vi "ClientAPI Tree.vi"   [LabVIEW 2020, in "CSM-TCP-Router.lvlib"]
uses:
  CSM-TCP-Router.lvlib
  TcpRouter-Client.lvclass
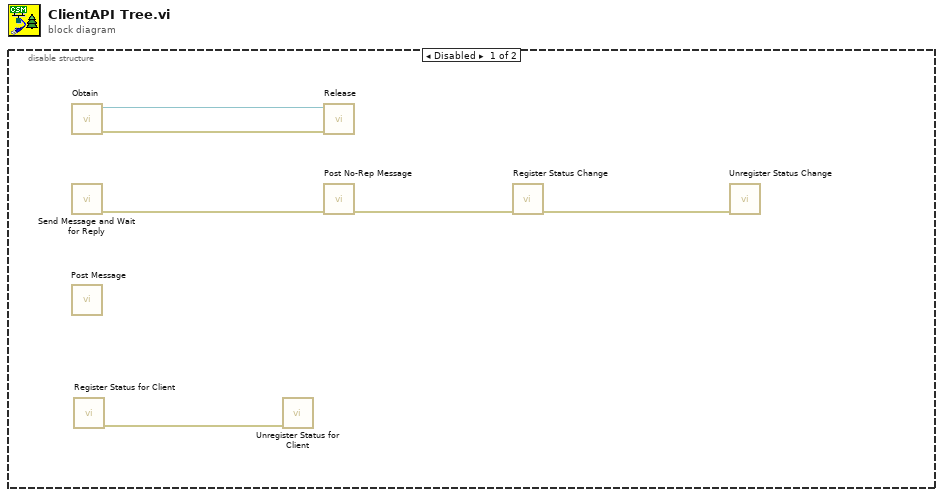
[diagram p0: block diagram]
diagram:
  n1 = disable-structure shown="Disabled" {
    frame Disabled {
      n2 = call "Obtain.vi"() -> ("error out"=w5:errorcluster, "TcpRouter-Client out"=w6:refnum<class "TcpRouter-Client.lvclass">)  [unwired: 10 in]
      n3 = call "Send Message and Wait for Reply.vi"() -> ("error out"=w4:errorcluster)  [unwired: 10 in, 1 out]
      n4 = call "Post Message.vi"() -> ()  [unwired: 11 in, 1 out]
      n5 = call "Register Status for Client.vi"() -> ("error out"=w2:errorcluster)  [unwired: 14 in, 1 out]
      n6 = call "Unregister Status for Client.vi"("error in (no error)"=w2) -> ()  [unwired: 13 in, 2 out]
      n7 = call "Release.vi"("error in (no error)"=w5, "TcpRouter-Client in"=w6) -> ()  [unwired: 9 in, 1 out]
      n8 = call "Post No-Rep Message.vi"("error in (no error)"=w4) -> ("error out"=w1:errorcluster)  [unwired: 10 in]
      n9 = call "Register Status Change.vi"("error in (no error)"=w1) -> ("error out"=w3:errorcluster)  [unwired: 13 in, 1 out]
      n10 = call "Unregister Status Change.vi"("error in (no error)"=w3) -> ()  [unwired: 13 in, 2 out]
    }
    frame Enabled {
    }
  }
